vi "Enable Disable Add Remove buttons.vi"(5 "Force add disabled (F)":bool, 7 "not present item indexes":i32[](array[numeric]), 8 "error in (no error)":errorcluster, 9 "selected items":i32[](array[numeric]), 10 "remove button":refnum<vi>, 11 "add button":refnum<vi>) -> (0 "error out":errorcluster)   [LabVIEW 2015, in "Engine Simulation Toolkit System Explorer.lvlib"]
uses:
  Engine Simulation Toolkit System Explorer.lvlib
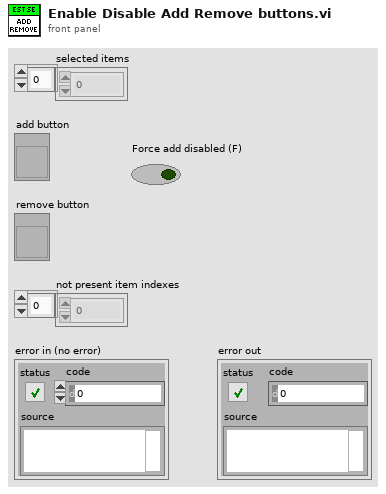
[diagram p1: front panel]
types:
  T1 = enum8{"Enabled", "Disabled", "Disabled and Grayed Out"}
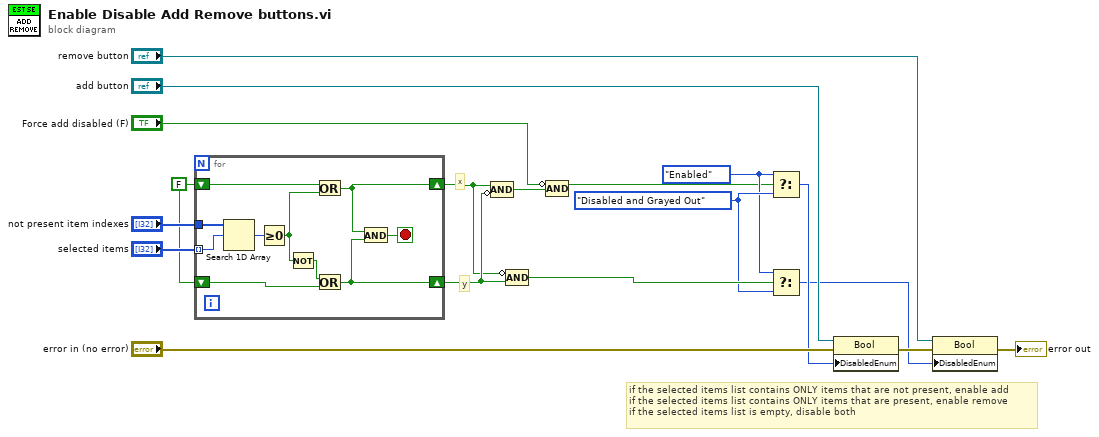
[diagram p0: block diagram]
diagram:
  w10 = FALSE
  w5 = T1."Disabled and Grayed Out" ("Disabled")
  w4 = T1."Enabled" ("Disabled")
  # "y"
  # "x"
  # "if the selected items list contains ONLY items that are not present, enable add\nif the selected items list contains ONLY items that are present, enable remove\nif the selected items list is empty, disable both"
  n1 = for {
    tunnel: "selected items" -> [w27] mode=indexing
    tunnel: "not present item indexes" -> [w28]
    shift-right: [w19] -> w7
    shift-left: w10 -> [w21]
    shift-right: [w22] -> w8
    shift-left: w10 -> [w24]
    stop <- w23 stop-if-true
    n2 = Search 1D Array(1D array=w28, element=w27) -> (index of element=w26:i32)  [unwired: 1 in]
    n3 = Greater Or Equal To 0?(x=w26) -> (x >= 0?=w20:bool)
    n4 = Not(x=w20) -> (.not. x?=w25:bool)
    n5 = Or(x=w21, y=w20) -> (x .or. y?=w19:bool)
    n6 = Or(x=w25, y=w24) -> (x .or. y?=w22:bool)
    n7 = And(x=w19, y=w22) -> (x .and. y?=w23:bool)
  }
  n8 = Compound Arithmetic op=AND(w7, invert w8) -> (w2:bool)
  n9 = Compound Arithmetic op=AND(invert w7, w8) -> (w6:bool)
  n10 = Compound Arithmetic op=AND(invert "Force add disabled (F)", w2) -> (w3:bool)
  n11 = Select(t=w4, s=w3, f=w5) -> (s? t:f=w11:T1)
  n12 = Select(t=w4, s=w6, f=w5) -> (s? t:f=w9:T1)
  n13 = property on="Property Node" class="Bool"(reference="add button", error in="error in (no error)", "DisabledEnum"=w11) -> (error out=w16:errorcluster)  [unwired: 1 out]
  n14 = property on="Property Node" class="Bool"(reference="remove button", error in=w16, "DisabledEnum"=w9) -> (error out=→"error out":errorcluster)  [unwired: 1 out]
